vi "exit_attempt2.vi"() -> ()   [LabVIEW 2015]
uses:
  <vilib>/LabVIEW Interface for Arduino/Type Defs/Board Type.ctl
  <vilib>/LabVIEW Interface for Arduino/Type Defs/Connection Type.ctl
  <vilib>/LabVIEW Interface for Arduino/Type Defs/Pin Mode.ctl
  <vilib>/LabVIEW Interface for Arduino/LabVIEW Interface for Arduino.lvlib
panel:
  out "Tab Control":T1(tab)
  out "?":string
  in  "Exit the program":bool
  in  "Start Test":bool
  in  "stop":bool
  in  "Lights":bool
  in  "Next Button 2":bool
  out "String 2":string
  in  "Next Button 3":bool
  out "String 3":string
  in  "Next Button 4":bool
  out "String 4":string
  in  "OK Button":bool
  out "Last  Message":string
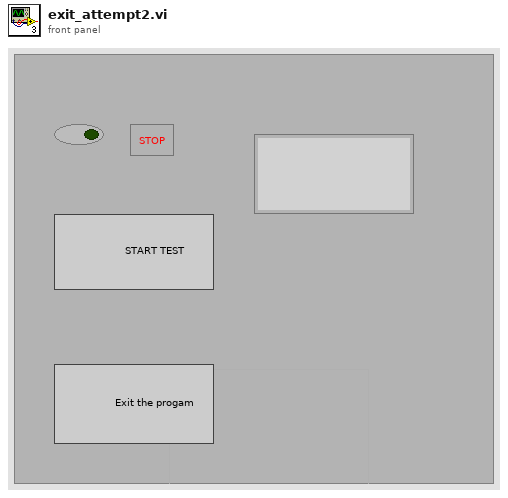
[diagram p1: front panel]
types:
  T1 = enum32{"Page 1", "Page 2", "Page 3", "Page 4", "Page 5"}
  T2 = typedef "LabVIEW Interface for Arduino.lvlib/Pin Mode.ctl" = enum8{"Input", "Output"}
  T3 = typedef "LabVIEW Interface for Arduino.lvlib/Connection Type.ctl" = enum8{"USB / Serial", "XBEE", "BlueSmirf (Bluetooth)"}
  T4 = typedef "LabVIEW Interface for Arduino.lvlib/Board Type.ctl" = enum16{"Uno", "Dimuelanove w/Atmega 328", "Mega 2560"}
  T5 = typedef "LabVIEW Interface for Arduino.lvlib/Arduino Resource.ctl" = cluster{"VISA resource":refnum<visa-resource-name>, "Board Type":T4, "Connection Type":enum8{"USB / Serial"}, "Bytes Per Packet (15)":u8}
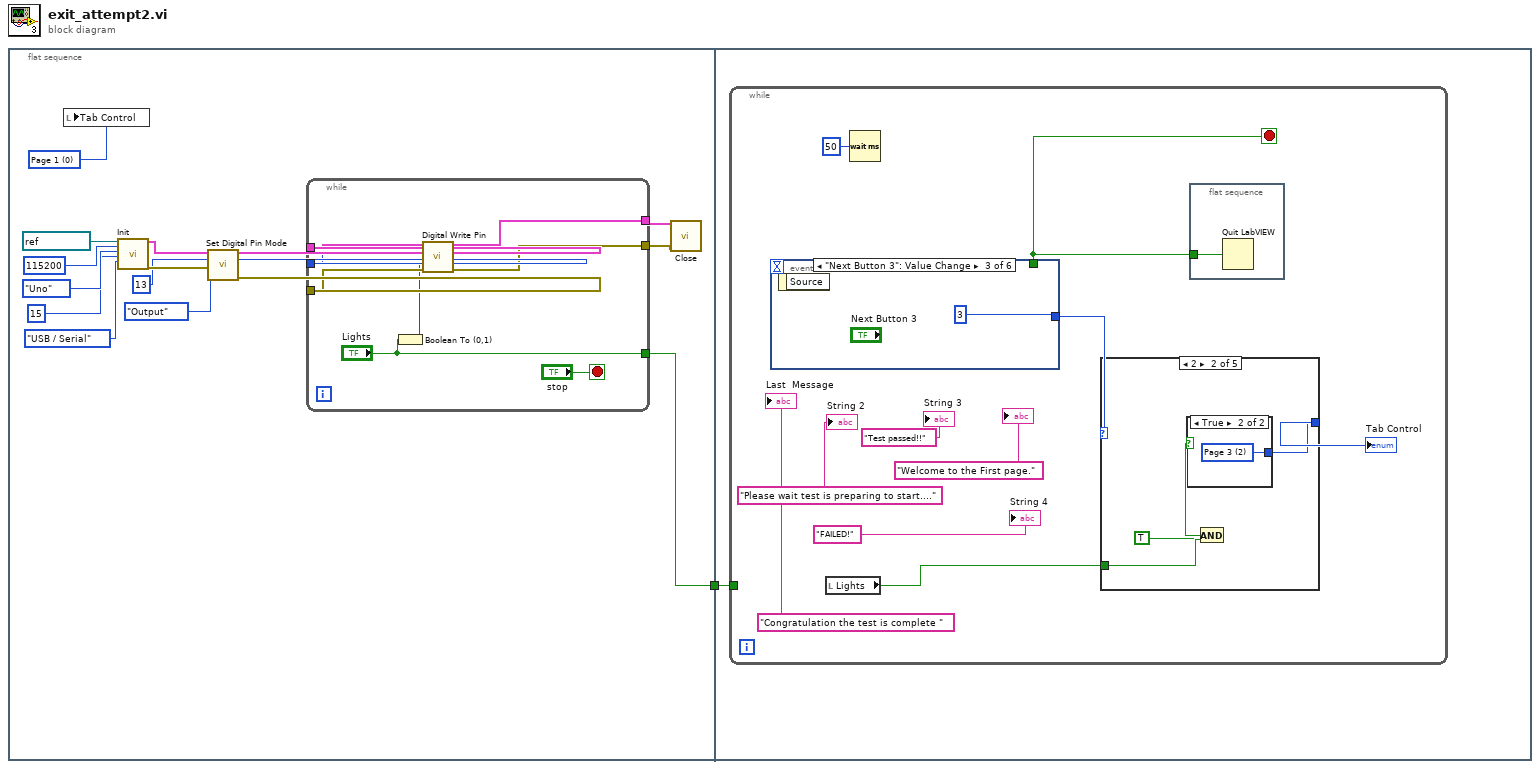
[diagram p0: block diagram]
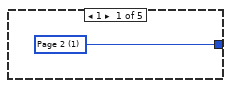
[diagram p2: hidden frame]
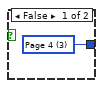
[diagram p3: hidden frame]
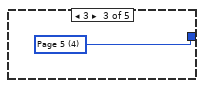
[diagram p4: hidden frame]
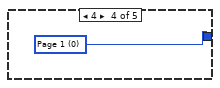
[diagram p5: hidden frame]
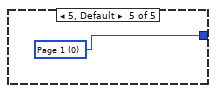
[diagram p6: hidden frame]
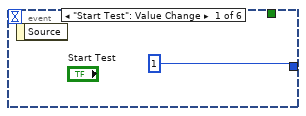
[diagram p7: hidden frame]
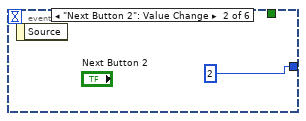
[diagram p8: hidden frame]
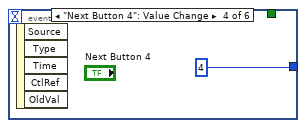
[diagram p9: hidden frame]
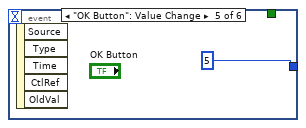
[diagram p10: hidden frame]
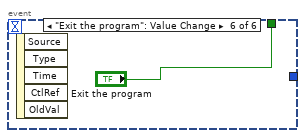
[diagram p11: hidden frame]
diagram:
  n1 = flat-sequence {
    tunnel: [w2] -> w1
    tunnel: w1 -> [w25]
    frame #0 {
      w5 = u8 13 ("Digital I/O Pin")
      w16 = u16 0 items=["Page 1"]
      n2 = local write "Tab Control"(w16) -> ()
      n3 = call <vilib>:"Init.vi"("VISA resource"=refnum<visa-resource-name> "COM73", "Baud Rate (115200)"=u32 115200, "Board Type (Uno)"=Board_Type."Uno", "Bytes Per Packet (15)"=u32 15, "Connection Type (USB/Serial)"=Connection_Type."USB / Serial") -> ("Arduino Resource"=w10:T5, "error out"=w9:errorcluster)  [unwired: 13 in]
      n4 = call <vilib>:"Set Digital Pin Mode.vi"("Arduino Resource"=w10, "Digital I/O Pin"=w5, "Pin Mode (Input)"=Pin_Mode."Output", "error in"=w9) -> ("Arduino Resource"=w7:T5, "error out"=w6:errorcluster)  [unwired: 10 in]
      n5 = while {
        tunnel: w7 -> [w24]
        tunnel: w6 -> [w23]
        tunnel: w5 -> [w20]
        tunnel: [w21] -> w4
        tunnel: [w19] -> w3
        tunnel: ["Lights"] -> w2
        stop <- "stop" stop-if-true
        n6 = Boolean To (0,1)(Boolean="Lights") -> (0, 1=w18:i16)
        n7 = call <vilib>:"Digital Write Pin.vi"("Arduino Resource"=w24, "Digital I/O Pin (0)"=w20, "Value (0)"=w18, "error in"=w23) -> ("Arduino Resource"=w21:T5, "error out"=w19:errorcluster)  [unwired: 10 in]
      }
      n8 = call <vilib>:"Close.vi"("Arduino Resource"=w4, "error in"=w3) -> ()  [unwired: 13 in, 1 out]
    }
    frame #1 {
      n9 = while {
        tunnel: w25 -> [_]
        stop <- w30 stop-if-true
        n10 = event shown="[2] \"Next Button 3\": Value Change" {
          selector: _ -> [_ _ _ _ _ _]
          dyn-events: _ -> [_ _ _ _ _ _]
          timeout: _ -> [_ _ _ _ _ _]
          tunnel: [1 2 3 4 5 _] -> w34
          tunnel: [_ _ _ _ _ "Exit the program"] -> w30
          event "Start Test": Value Change {
            n11 = event-data() -> ()  [unwired: 1 in, 1 out]
          }
          event "Next Button 2": Value Change {
            n12 = event-data() -> ()  [unwired: 1 in, 1 out]
          }
          event "Next Button 3": Value Change {
            n13 = event-data() -> ()  [unwired: 1 in, 1 out]
          }
          event "Next Button 4": Value Change {
            n14 = event-data() -> ()  [unwired: 1 in, 5 out]
          }
          event "OK Button": Value Change {
            n15 = event-data() -> ()  [unwired: 1 in, 5 out]
          }
          event "Exit the program": Value Change {
            n16 = event-data() -> ()  [unwired: 1 in, 5 out]
          }
        }
        n17 = local read "Lights"() -> (w27:bool)
        n18 = Wait (ms)(milliseconds to wait=u32 50) -> ()  [unwired: 1 out]
        n19 = case shown="2" w34 {
          tunnel: [w36 w38 w43 w44 w45] -> w28
          tunnel: w27 -> [_ w40 _ _ _]
          frame 1 {
            w36 = u16 1 items=["Page 1", "Page 2", "Page 3"]
          }
          frame 2 {
            n20 = And(x=TRUE, y=w40) -> (x .and. y?=w37:bool)
            n21 = case shown="True" w37 {
              tunnel: [w41 w42] -> w38
              frame False {
                w41 = u16 3 items=["Page 1", "Page 2", "Page 3", "Page 4"]
              }
              frame True {
                w42 = u16 2 items=["Page 1", "Page 2", "Page 3", "Page 4"]
              }
            }
          }
          frame 3 {
            w43 = u16 4 items=["Page 1", "Page 2", "Page 3", "Page 4", "Page 5"]
          }
          frame 4 {
            w44 = u16 0 items=["Page 1"]
          }
          frame 5, Default {
            w45 = u16 0 items=["Page 1"]
          }
        }
        "Tab Control" <- w28
        n22 = flat-sequence {
          tunnel: w30 -> [w52]
          frame #0 {
            n23 = Quit LabVIEW(quit? (T)=w52) -> ()
          }
        }
        "?" <- "Welcome to the First page."
        "String 2" <- "Please wait test is preparing to start...."
        "String 3" <- "Test passed!!"
        "String 4" <- "FAILED!"
        "Last  Message" <- "Congratulation the test is complete "
      }
    }
  }
